vi "表格文件.vi"() -> ()   [LabVIEW 2014]
uses:
  <vilib>/Utility/file.llb/Write To Spreadsheet File (DBL).vi
panel:
  in  "开始写入":bool
  in  "是否转置":bool
  in  "是否写入文件":bool
  in  "数组":dbl[](array[numeric])
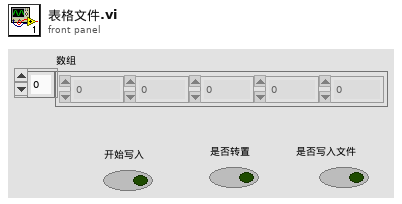
[diagram p1: front panel]
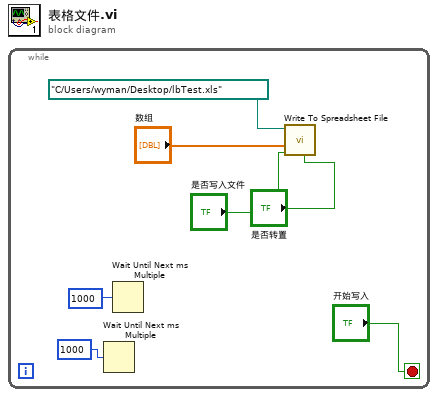
[diagram p0: block diagram]
diagram:
  n1 = while {
    stop <- "开始写入" stop-if-true
    n2 = Wait Until Next ms Multiple(millisecond multiple=1000) -> ()  [unwired: 1 out]
    n3 = Wait Until Next ms Multiple(millisecond multiple=1000) -> ()  [unwired: 1 out]
    n4 = call-poly <vilib>:"Write To Spreadsheet File.vi"("transpose? (no:F)"="是否转置", "append to file? (new file:F)"="是否写入文件", "1D data"="数组", "file path (dialog if empty)"=path "C:/Users/wyman/Desktop/lbTest.xls") -> ()  [unwired: 4 in, 1 out]
  }
